vi "New_Magazine_Begin.vi"   [LabVIEW 2019]
uses:
  New_Magazine_Cluster.ctl
  New_Magazine_Control_States.ctl
  New_Magazine_Globals.vi
types:
  T1 = typedef "New_Magazine_Cluster.ctl" = cluster{"Control_States":T2, "Firing":bool, "Throttle":dbl, "Spinning Up":bool, "Off":bool}
  T2 = typedef "New_Magazine_Control_States.ctl" = enum16{"No-Op", "Up", "Down", "Manual", "Fire", "Spinning Up"}
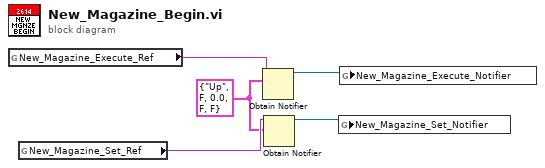
[diagram p0: block diagram]
diagram:
  w1 = T1 {"Control_States"=enum."Up", "Firing"=FALSE, "Throttle"=0.0, "Spinning Up"=FALSE, "Off"=FALSE}
  n1 = global read "New_Magazine_Globals.vi" "New_Magazine_Execute_Ref"() -> (w2:string)
  n2 = global read "New_Magazine_Globals.vi" "New_Magazine_Set_Ref"() -> (w3:string)
  n3 = Obtain Notifier(name (unnamed)=w2, notification data type=w1) -> (notifier out=w4:refnum<notifier>)  [unwired: 2 in, 2 out]
  n4 = Obtain Notifier(name (unnamed)=w3, notification data type=w1) -> (notifier out=w5:refnum<notifier>)  [unwired: 2 in, 2 out]
  n5 = global write "New_Magazine_Globals.vi" "New_Magazine_Set_Notifier"(w5) -> ()
  n6 = global write "New_Magazine_Globals.vi" "New_Magazine_Execute_Notifier"(w4) -> ()
